vi "FormVarValuesArray.vi"(2 "varables bytes":i32[](array[numeric]), 3 "varables ports":i32[](array[numeric]), 4 "Ports":u8[](array[numeric])) -> (1 "Values Array":string[](array[string]))   [LabVIEW 2019]
panel:
  out "Boolean array":bool[](array[boolean])
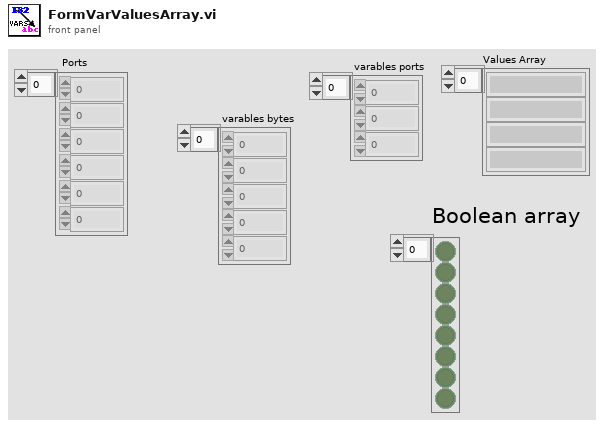
[diagram p1: front panel]
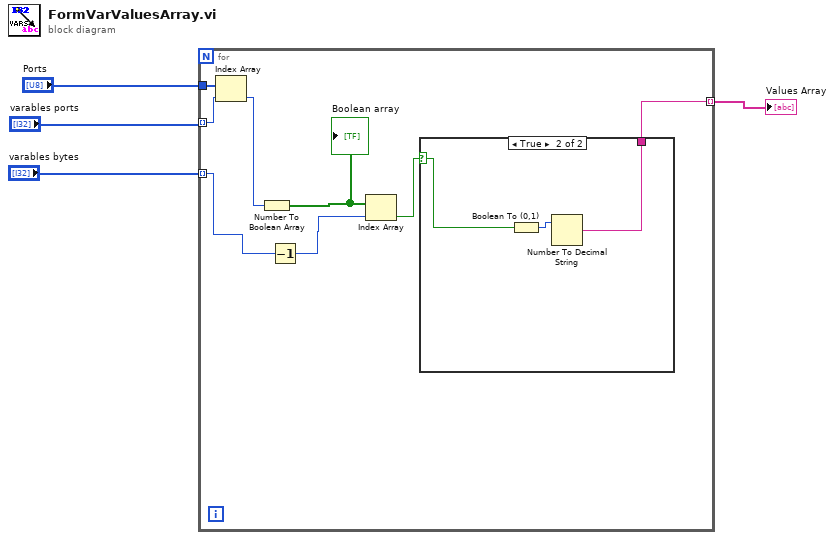
[diagram p0: block diagram]
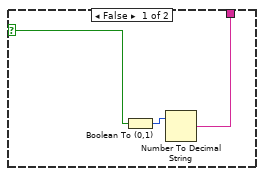
[diagram p2: hidden frame]
diagram:
  n1 = for {
    tunnel: "varables ports" -> [w11] mode=indexing
    tunnel: "Ports" -> [w12]
    tunnel: "varables bytes" -> [w6] mode=indexing
    tunnel: [w10] -> w1 mode=indexing
    n2 = Index Array(array=w12, index=w11) -> (element=w7:u8)
    n3 = Number To Boolean Array(number=w7) -> (Boolean array=w9:bool[])
    "Boolean array" <- w9
    n4 = Decrement(x=w6) -> (x-1=w5:i32)
    n5 = Index Array(array=w9, index=w5) -> (element=w8:bool)
    n6 = case shown="True" w8 {
      selector: w8 -> [w13 w16]
      tunnel: [w14 w17] -> w10
      frame False {
        n7 = Boolean To (0,1)(Boolean=w13) -> (0, 1=w15:i16)
        n8 = Number To Decimal String(number=w15) -> (decimal integer string=w14:string)  [unwired: 1 in]
      }
      frame True {
        n9 = Boolean To (0,1)(Boolean=w16) -> (0, 1=w18:i16)
        n10 = Number To Decimal String(number=w18) -> (decimal integer string=w17:string)  [unwired: 1 in]
      }
    }
  }
  "Values Array" <- w1
